vi "LuaVIEW Register Public Function.vi"(7 "function VI path":path, 11 "error in (no error)":errorcluster) -> (15 "error out":errorcluster)   [LabVIEW 2012]
doc: "Open a reference to a LuaVIEW function VI and add it to the public registry. Any LuaVIEW states that are opened after the function was registered will be able to call the function (unless \"Use Public Registry?\" was reset to false on opening the state). If the function VI was already registered, no further resources will be allocated."
uses:
  typedefs/t_LuaVIEW Daemon Exchange Methods.ctl
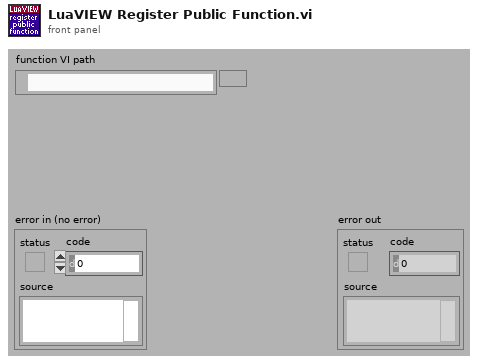
[diagram p1: front panel]
types:
  T1 = typedef "t_LuaVIEW Daemon Exchange Methods.ctl" = enum16{"inert", "send path", "send cleanup", "get sent", "reply", "get reply", "unset launched"}
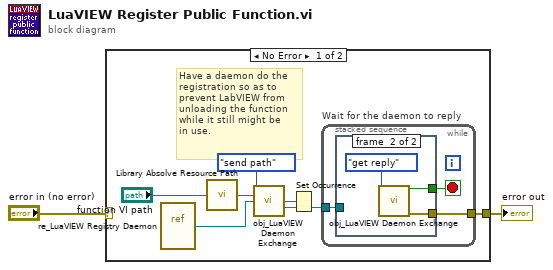
[diagram p0: block diagram]
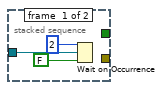
[diagram p2: hidden frame]
diagram:
  n1 = case shown="No Error" "error in (no error)" {
    selector: "error in (no error)" -> [_ w19]
    tunnel: [w6 w19] -> w2
    frame No Error {
      # "Have a daemon do the\nregistration so as to\nprevent LabVIEW from\nunloading the function\nwhile it still might be\nin use."
      n2 = vi-ref "re_LuaVIEW Registry Daemon.vi"() -> ("vi reference"=w3:refnum<vi>)
      n3 = call "Library Absolve Resource Path.vi"("path in"="function VI path") -> ("absolved path"=w4:path)  [unwired: 14 in]
      n4 = call "obj_LuaVIEW Daemon Exchange.vi"("method"=t_LuaVIEW_Daemon_Exchange_Methods."send path", "path in"=w4, "static daemon reference {send path}"=w3) -> ("send occurrence"=w7:refnum<k4>, "reply occurrence"=w8:refnum<k4>)  [unwired: 8 in, 3 out]
      n5 = Set Occurrence(w7) -> ()
      n6 = while "Wait for the daemon to reply" {
        tunnel: w8 -> [w12]
        tunnel: [w10] -> w6
        stop <- w11 stop-if-true
        n7 = stacked-sequence {
          tunnel: w12 -> [w15 _]
          tunnel: [_ w17] -> w11
          tunnel: [_ w16] -> w10
          frame #0 {
            n8 = Wait on Occurrence(1:FALSE ("ignore previous (T)"), 2:w15, 3:2 ("ms timeout (-1)")) -> ()  [unwired: 1 out]
          }
          frame #1 {
            n9 = call "obj_LuaVIEW Daemon Exchange.vi"("method"=t_LuaVIEW_Daemon_Exchange_Methods."get reply") -> ("available?"=w17:bool, "error reply out"=w16:errorcluster)  [unwired: 10 in, 3 out]
          }
        }
      }
    }
    frame Error {
    }
  }
  "error out" <- w2
